vi "Connect Subpanel to Manager.vi"(7 "Connect":bool, 8 "error in (no error)":errorcluster, 10 "Manager Port":u16, 11 "CIF_UI in":refnum<class "CIF_UI.lvclass">) -> (3 "CIF_UI out":refnum<class "CIF_UI.lvclass">)   [LabVIEW 2021, in "CIF_UI.lvclass"]
doc: "If a subpanel needs to directly communicate with the manager this will attempt to establish the connection. \nThe default value is to not connect. \nIf a port is provided it will override the manager port provided to the class. The default is 0 (no override)"
uses:
  CIF_UI.lvclass
  CIF_UI.lvclass/CIF_UI.ctl
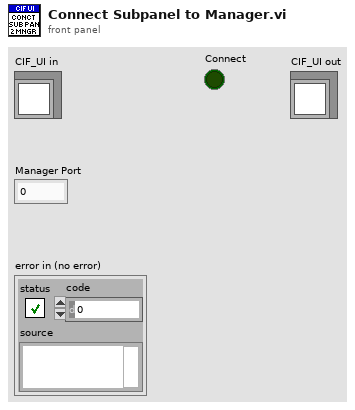
[diagram p1: front panel]
types:
  T1 = typedef "grpc-lvsupport-release.lvlib/grpcId.ctl" = u64
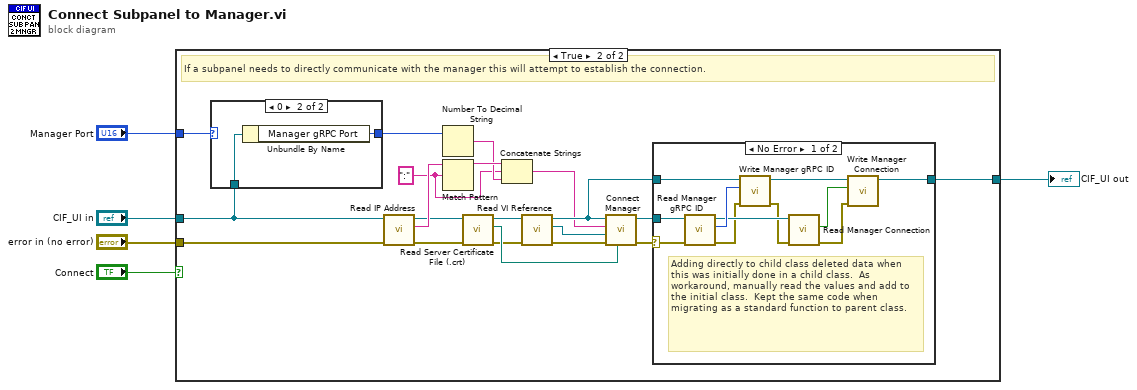
[diagram p0: block diagram]
diagram:
  n1 = case shown="True" "Connect" {
    tunnel: "error in (no error)" -> [_ w26]
    tunnel: "CIF_UI in" -> [w6 w9]
    tunnel: [w6 w14] -> w3
    tunnel: "Manager Port" -> [_ w7]
    frame False {
      # "Connection not needed.  Skip."
    }
    frame True {
      w10 = ":" ("regular expression")
      # "If a subpanel needs to directly communicate with the manager this will attempt to establish the connection."
      n2 = case shown="0" w7 {
        selector: w7 -> [w27 _]
        tunnel: w9 -> [_ w29]
        tunnel: [w27 w28] -> w8
        frame 1, Default {
        }
        frame 0 {
          n3 = Unbundle By Name(w29) -> ("Manager gRPC Port"=w28:u16)
        }
      }
      n4 = call "Read IP Address.vi"("error in (no error)"=w26, "CIF_UI in"=w9) -> ("error out"=w22:errorcluster, "IP address"=w25:string, "CIF_UI out"=w23:refnum<class "CIF_UI.lvclass">)  [unwired: 7 in]
      n5 = Number To Decimal String(number=w8) -> (decimal integer string=w11:string)  [unwired: 1 in]
      n6 = Match Pattern(string=w25, regular expression=w10) -> (before substring=w12:string)  [unwired: 1 in, 3 out]
      n7 = call "Read Server Certificate File (.crt).vi"("error in (no error)"=w22, "CIF_UI in"=w23) -> ("error out"=w20:errorcluster, "Server Certificate File (.crt)"=w24:path, "CIF_UI out"=w21:refnum<class "CIF_UI.lvclass">)  [unwired: 7 in]
      n8 = Concatenate Strings(w12, w10, w11) -> (w13:string)
      n9 = call "Read VI Reference.vi"("error in (no error)"=w20, "CIF_UI in"=w21) -> ("error out"=w19:errorcluster, "VI Reference"=w18:refnum<vi>, "CIF_UI out"=w16:refnum<class "CIF_UI.lvclass">)  [unwired: 7 in]
      n10 = call "Connect Manager.vi"("Server Certificate File (.crt)"=w24, "error in (no error)"=w19, "VI Reference"=w18, "Address"=w13, "CIF_UI in"=w16) -> ("error out"=w17:errorcluster, "CIF_UI out"=w15:refnum<class "CIF_UI.lvclass">)  [unwired: 5 in]
      n11 = case shown="No Error" w17 {
        selector: w17 -> [w39 _]
        tunnel: w15 -> [w40 _]
        tunnel: [w30 w41] -> w14
        tunnel: w16 -> [w38 w41]
        frame No Error {
          # "Adding directly to child class deleted data when this was initially done in a child class.  As workaround, manually read the values and add to the initial class.  Kept the same code when migrating as a standard function to parent class."
          n12 = call "Read Manager gRPC ID.vi"("error in (no error)"=w39, "CIF_UI in"=w40) -> ("error out"=w35:errorcluster, "Manager gRPCid"=w37:T1, "CIF_UI out"=w36:refnum<class "CIF_UI.lvclass">)  [unwired: 7 in]
          n13 = call "Write Manager gRPC ID.vi"("error in (no error)"=w35, "gRPCid"=w37, "CIF_UI in"=w38) -> ("error out"=w34:errorcluster, "CIF_UI out"=w33:refnum<class "CIF_UI.lvclass">)  [unwired: 7 in]
          n14 = call "Read Manager Connection.vi"("error in (no error)"=w34, "CIF_UI in"=w36) -> ("error out"=w32:errorcluster, "Manager Connection"=w31:bool)  [unwired: 7 in, 1 out]
          n15 = call "Write Manager Connection.vi"("error in (no error)"=w32, "Manager Connection"=w31, "CIF_UI in"=w33) -> ("CIF_UI out"=w30:refnum<class "CIF_UI.lvclass">)  [unwired: 7 in, 1 out]
        }
        frame Error {
        }
      }
    }
  }
  "CIF_UI out" <- w3
